vi "Error Module.vi"(7 "Error Module Command":T4=enum."Handle Errors", 8 "error in (no error)":errorcluster, 9 "User Event Reference":T1, 10 "Display Queue Reference":T2, 11 "Consumer Control Reference":T3) -> (0 "error out":errorcluster)   [LabVIEW 2021]
uses:
  Controls/Error Module Command.ctl
  Controls/Consumer Control Reference.ctl
  Controls/Consumer Control.ctl
  Controls/Display Queue Reference.ctl
  Controls/Display and Datalog Control.ctl
  Controls/User Event Reference.ctl
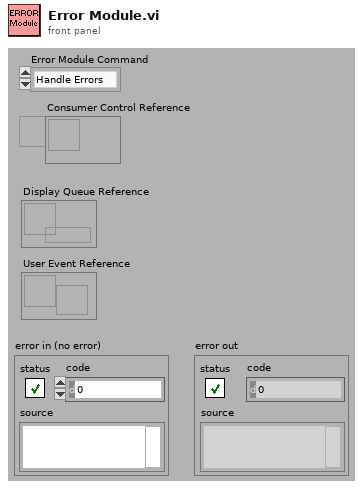
[diagram p1: front panel]
types:
  T1 = typedef "User Event Reference.ctl" = refnum<user-event>
  T2 = typedef "Display Queue Reference.ctl" = refnum<queue>
  T3 = typedef "Consumer Control Reference.ctl" = refnum<queue>
  T4 = typedef "Error Module Command.ctl" = enum16{"Initialize", "Handle Errors", "Report Errors"}
  T5 = typedef "Display and Datalog Control.ctl" = cluster{"Command":enum16{"Initialize", "Initialize Display", "Update Data", "Update Progress", "Exit"}, "Data":variant}
  T6 = typedef "Consumer Control.ctl" = cluster{"Command":enum16{"Initialize", "Home", "Configure Channels", "Fixed Range", "Set DC Supply", "Save Settings", "Load Settings", "Power Test", "Power Test M", "Run Configuration", "Run Test", "Abort", "Run EQ", "Check EQ", "Help", "Exit"}, "Data":variant}
  T7 = typedef "ctl_Display Queue Reference.ctl" = refnum<queue>
  T8 = typedef "ctl_User Event Reference.ctl" = refnum<user-event>
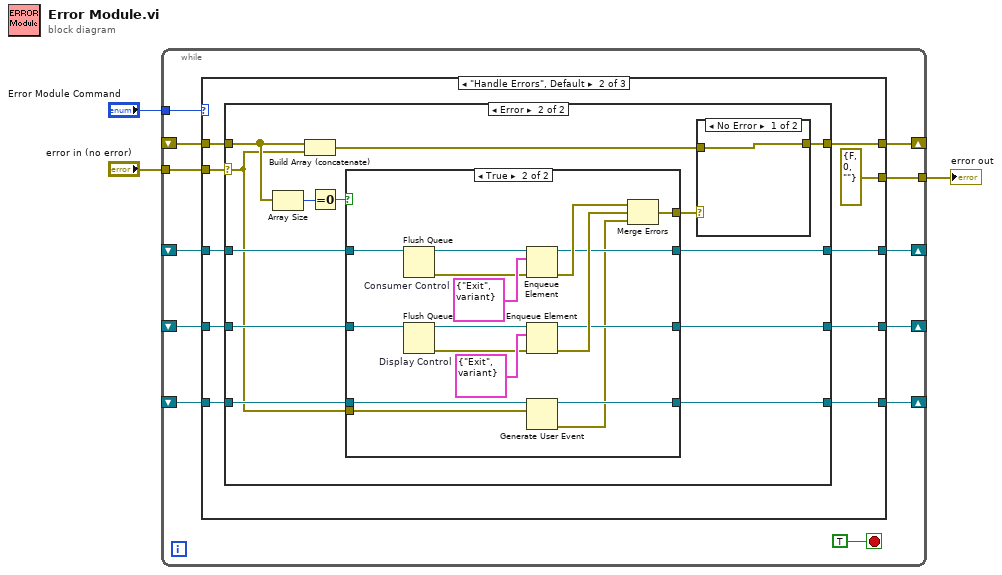
[diagram p0: block diagram]
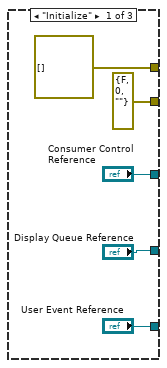
[diagram p2: hidden frame]
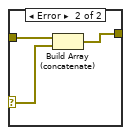
[diagram p4: hidden frame]
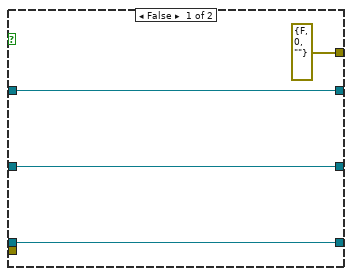
[diagram p5: hidden frame]
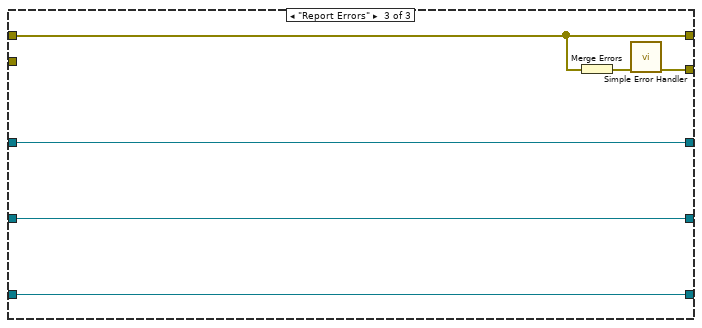
[diagram p6: hidden frame]
diagram:
  n1 = while {
    tunnel: "Error Module Command" -> [w15]
    tunnel: "error in (no error)" -> [w14]
    tunnel: [w13] -> w1
    shift-right: [w12] -> _
    shift-left: _ -> [w9]
    shift-right: [w11] -> _
    shift-left: _ -> [w8]
    shift-right: [w10] -> _
    shift-left: _ -> [w7]
    shift-right: [w6] -> _
    shift-left: _ -> [w5]
    stop <- TRUE stop-if-true
    n2 = case shown="\"Handle Errors\", Default" w15 {
      tunnel: w14 -> [_ w30 _]
      tunnel: [errorcluster {"status"=FALSE, "code"=0, "source"=""} ("error out") errorcluster {"status"=FALSE, "code"=0, "source"=""} ("error out") w73] -> w13
      tunnel: ["Consumer Control Reference" w24 w77] -> w12
      tunnel: ["Display Queue Reference" w25 w76] -> w11
      tunnel: ["User Event Reference" w26 w75] -> w10
      tunnel: w9 -> [_ w29 w77]
      tunnel: w8 -> [_ w28 w76]
      tunnel: w7 -> [_ w27 w75]
      tunnel: [errorcluster[] [] w23 w78] -> w6
      tunnel: w5 -> [_ w22 w78]
      frame "Initialize" {
      }
      frame "Handle Errors", Default {
        n3 = case shown="Error" w30 {
          selector: w30 -> [_ w39]
          tunnel: [w34 w42] -> w24
          tunnel: w29 -> [w34 w44]
          tunnel: [w33 w41] -> w25
          tunnel: w28 -> [w33 w43]
          tunnel: [w32 w38] -> w26
          tunnel: w27 -> [w32 w40]
          tunnel: [w31 w36] -> w23
          tunnel: w22 -> [w31 w47]
          frame No Error {
          }
          frame Error {
            n4 = Array Size(array=w47) -> (size(s)=w46:i32)
            n5 = Build Array (concatenate)(w47, w39) -> (w35:errorcluster[])
            n6 = Equal To 0?(x=w46) -> (x = 0?=w45:bool)
            n7 = case shown="True" w45 {
              tunnel: w44 -> [w54 w72]
              tunnel: w43 -> [w53 w71]
              tunnel: [w54 w62] -> w42
              tunnel: [w53 w61] -> w41
              tunnel: w40 -> [w52 w60]
              tunnel: w39 -> [_ w58]
              tunnel: [w52 w59] -> w38
              tunnel: [errorcluster {"status"=FALSE, "code"=0, "source"=""} ("error out") w56] -> w37
              frame False {
              }
              frame True {
                w66 = T5 {"Command"=enum."Exit", "Data"=variant}  # Display Control
                w68 = T6 {"Command"=enum."Exit", "Data"=variant}  # Consumer Control
                n8 = Flush Queue(queue=w72) -> (queue out=w70:T3, error out=w67:errorcluster)  [unwired: 1 in, 1 out]
                n9 = Flush Queue(queue=w71) -> (queue out=w69:T7, error out=w65:errorcluster)  [unwired: 1 in, 1 out]
                n10 = Enqueue Element(queue=w70, element=w68, error in (no error)=w67) -> (queue out=w62:T3, error out=w64:errorcluster)  [unwired: 1 in, 1 out]
                n11 = Enqueue Element(queue=w69, element=w66, error in (no error)=w65) -> (queue out=w61:T7, error out=w63:errorcluster)  [unwired: 1 in, 1 out]
                n12 = Generate User Event(user event=w60, event data cluster=w58) -> (user event out=w59:T8, error out=w57:errorcluster)  [unwired: 2 in]
                n13 = Merge Errors(w64, w63, w57) -> (w56:errorcluster)
              }
            }
            n14 = case shown="No Error" w37 {
              selector: w37 -> [_ w51]
              tunnel: [w48 w49] -> w36
              tunnel: w35 -> [w48 w50]
              frame No Error {
              }
              frame Error {
                n15 = Build Array (concatenate)(w50, w51) -> (w49:errorcluster[])
              }
            }
          }
        }
      }
      frame "Report Errors" {
        n16 = Merge Errors(w78) -> (w74:errorcluster)
        n17 = call <vilib>:"Simple Error Handler.vi"("error in (no error)"=w74) -> ("error out"=w73:errorcluster)  [unwired: 4 in, 4 out]
      }
    }
  }
  "error out" <- w1
